vi "ble_evt_connection_disconnected.vi"(8 "error in (no error)":errorcluster, 11 "COM Bluegiga in":refnum<visa-resource-name>) -> (0 "error out":errorcluster, 3 "COM Bluegiga out":refnum<visa-resource-name>)   [LabVIEW 2015]
uses:
  type_def/message_class.ctl
  type_def/message_type.ctl
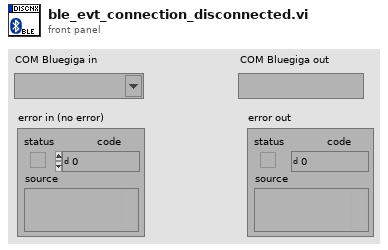
[diagram p1: front panel]
types:
  T1 = typedef "message_type.ctl" = u8
  T2 = typedef "message_class.ctl" = u8
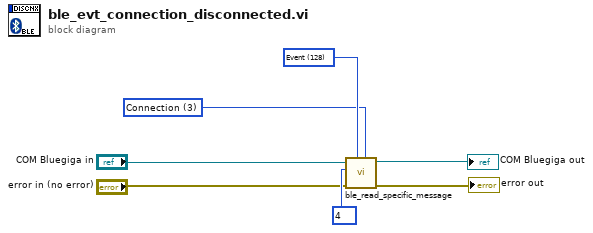
[diagram p0: block diagram]
diagram:
  w5 = T1 128 items=["Command / Response"=0, "Event"=128] ("Message Type (Response)")
  w4 = T2 3 items=["System", "Persistent Store", "Attribute database", "Connection", "Attribute client", "Security Manager", "Generic Access Profile", "Hardware"] ("Command Class (System)")
  n1 = call "ble_read_specific_message.vi"("Command Class (System)"=w4, "Message Type (Response)"=w5, "error in (no error)"="error in (no error)", "Message ID (0x00)"=u8 4, "COM Bluegiga in"="COM Bluegiga in") -> ("error out"=→"error out":errorcluster, "COM Bluegiga out"=→"COM Bluegiga out":refnum<visa-resource-name>)  [unwired: 2 in, 3 out]
